vi "Invalid INI Read.vi"(8 "error in":errorcluster, 11 "Editor Position in":refnum<class "Editor Position.lvclass">) -> (0 "error out":errorcluster, 3 "Editor Position out":refnum<class "Editor Position.lvclass">)   [LabVIEW 2021, in "Editor Position.lvclass"]
doc: "Tests reading an invalidly formated data in the position key."
uses:
  Editor Position.lvclass
  C:/Program Files/National Instruments/LabVIEW 2024/vi.lib/Astemes/LUnit/Test Case.lvclass
  <vilib>/Utility/miscctls.llb/LVRectTypeDef.ctl
  <vilib>/Astemes/LUnit/Test Case.lvclass/Test Case.ctl
  c60327dd-cdad-4b8c-8243-7f44ee2244ce.vi
  <vilib>/Astemes/LUnit/Core/LUnit Test Case/Private/Append Pass Result.vi
  <vilib>/Astemes/LUnit/Core/LUnit Test Case/Private/Append Fail Result.vi
  c60327dd-cdad-4b8c-8243-7f44ee2244ce.vi/9c5d11cd-9439-4240-a1ee-d9baace9c924.vi
  <vilib>/Astemes/LUnit/Core/LUnit Test Case/Private/Run In UI.vi
  <vilib>/Utility/error.llb/Clear Errors.vi
  <resource>/dialog/lvconfig.llb/LV Config Write String.vi
  <vilib>/LabVIEW Icon API/lv_icon/lv_icon.lvlib
  <vilib>/Astemes/LUnit/Test Case.lvclass
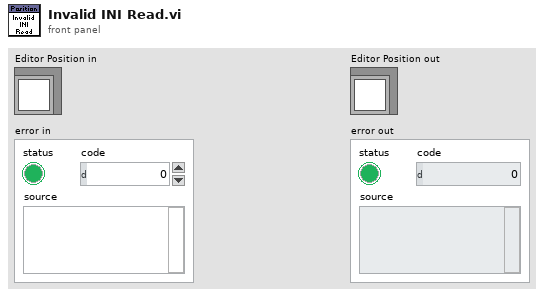
[diagram p1: front panel]
types:
  T1 = typedef "LVRectTypeDef.ctl" = cluster{"Left":i16, "Top":i16, "Right":i16, "Bottom":i16}
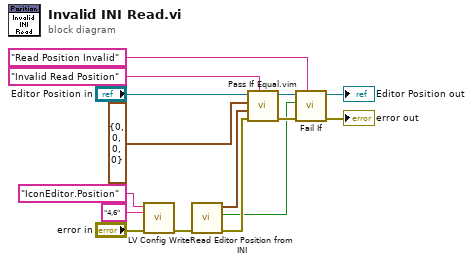
[diagram p0: block diagram]
diagram:
  n1 = call-poly <resource>:"LV Config Write.vi"("error in (no error)"="error in", "value"="4,6", "key"="IconEditor.Position") -> ("error out"=w11:errorcluster)  [unwired: 4 in]
  n2 = call <resource>:"Read Editor Position from INI.vi"("error in"=w11) -> ("error out"=w14:errorcluster, "Bounds Valid"=w5:bool, "Window Bounds"=w6:T1)  [unwired: 7 in, 1 out]
  n3 = call "Pass If Equal.vim"("Description"="Invalid Read Position", "error in (no error)"=w14, "Actual"=w6, "Expected"=T1 {"Left"=0, "Top"=0, "Right"=0, "Bottom"=0} ("Window Bounds"), "LUnit Test Case In"="Editor Position in") -> ("error out"=w15:errorcluster, "LUnit Test Case Out"=w10:refnum<class "Editor Position.lvclass">)  [unwired: 5 in]
  n4 = call <vilib>:"Fail If.vi"("Description"="Read Position Invalid", "error in (no error)"=w15, "Fail?"=w5, "LUnit Test Case In"=w10) -> ("error out"=→"error out":errorcluster, "LUnit Test Case Out"=→"Editor Position out":refnum<class "Editor Position.lvclass">)  [unwired: 6 in]
